vi "5.11-OCU TCP Data Client.vi"() -> ()   [LabVIEW 2010]
doc: "Displays data sent via TCP from Data Server.vi. Once a TCP connection is open, the VI reads 4 bytes to determine the amount of data being sent. It then reads and charts that many bytes. If an error occurs or the stop button is pressed, it sends a \"Q\" to the Data Sender to notify it to quit.\n\n<B>Note:</B> Requires the Data Server.vi located in the same library as this VI."
uses:
  6-OCU Neurons/6.0-OCU to Forebrain Neuron.ctl
  6-OCU Neurons/6.1-Act.ctl
  6-OCU Neurons/6.1-UDP Saitek.ctl
  7-OCU/7.3-Mission Def/7.6 - GPS Waypoint Def.ctl
  6-OCU Neurons/MDF Array LatLong.ctl
  6-OCU Neurons/MDF LatLong.ctl
  5.0-Global.vi
panel:
  in  "Port":u16=22234 min=1025 step=1
  # "Instructions:\n1. Open the Data Server.vi located in the same library.\n2. Follow the instructions on it's front panel.\n\nNote: This VI is built to work with the Data Server.vi."
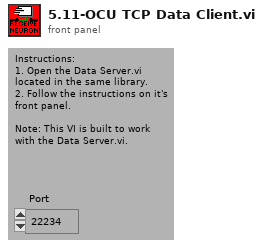
[diagram p1: front panel]
types:
  T1 = typedef "6.0-OCU to Forebrain Neuron.ctl" = cluster{"6.1 Act":T2, "7.6 - GPS Waypoints Data":T4}
  T2 = typedef "6.1-Act.ctl" = cluster{"6.1-Saitek Controller":T3, "Joystick Mode":bool, "Shutdown":bool, "Reset":bool, "Begin":bool}
  T3 = typedef "6.1-UDP Saitek.ctl" = cluster{"Stop":bool, "Setpoint":bool, "Run":bool, "Restart":bool, "Shutdown":bool, "Joystick\nMode 1":bool, "Joystick\nMode 2":bool, "Joystick \nMode 3":bool, "Joystick Mode 4":bool, "10":bool, "11":bool, "Pitch":sgl, "Roll":sgl, "Yaw":sgl, "Left":sgl, "Right":sgl}
  T4 = typedef "7.6 - GPS Waypoint Def.ctl" = cluster{"GPS Waypoint Center (Lat, Long)":dbl[], "5.1.1 MDF GPS":T5}
  T5 = typedef "MDF Array LatLong.ctl" = T6[]
  T6 = typedef "MDF LatLong.ctl" = cluster{"Waypoint #":dbl, "Latitude (waypoint)":ext, "Longitude  (waypoint)":ext}
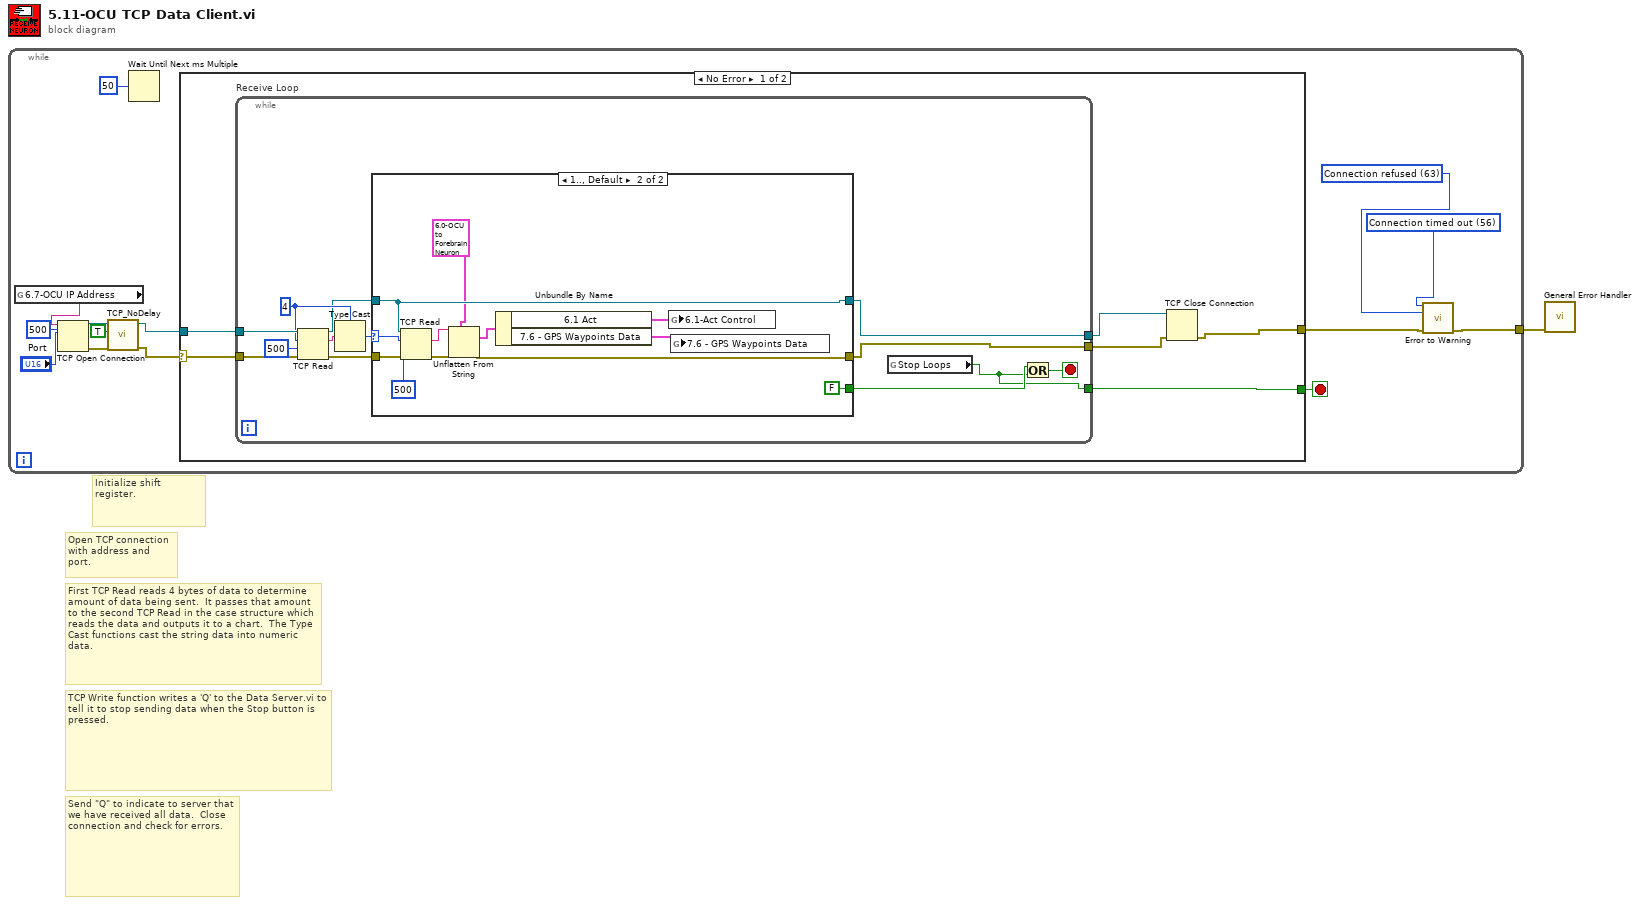
[diagram p0: block diagram]
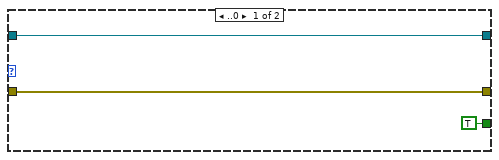
[diagram p2: hidden frame]
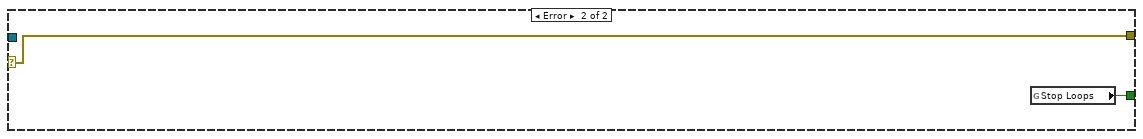
[diagram p3: hidden frame]
diagram:
  # "Initialize shift register."
  # "Send \"Q\" to indicate to server that we have received all data.  Close connection and check for errors."
  # "TCP Write function writes a 'Q' to the Data Server.vi to tell it to stop sending data when the Stop button is pressed."
  # "First TCP Read reads 4 bytes of data to determine amount of data being sent.  It passes that amount to the second TCP Read in the case structure which reads the data and outputs it to a chart.  The Type Cast functions cast the string data into numeric data."
  # "Open TCP connection with address and port."
  n1 = while {
    tunnel: [w5] -> w1
    stop <- w14 stop-if-true
    w3 = 63 items=["No Error", "Argument Error", "Memory Full", "Out of Zone", "End of File", "File Already Open", "Generic File IO Error", "File Not Found", "File Permission Error", "Disk Full", "Duplicate Path", "Too Many Files Open", "Not Enabled", "Resource File Not Found", "Cannot Add Resource", "Resource Not Found", "Image Not Found", "Image Memory Error", "Pen Does Not Exist", "Config Bad Type", "Config Token Not Found", "Config Parse Error", "Config Memory Error", "Bad External Code Format", "Bad External Code Offset", "External Code Not Present", "Null Window", "Destroy Window Mixup", "Null Menu", "Print Aborted", "Bad Print Record", "Print Driver Error", "Windows Error During Print", "Memory Error During Print", "Print Dialog Error", "Generic Print Error", "Invalid Device Refnum", "Device Not Found", "Device Parameter Error", "Device Unit Error", "Can't Open Device", "Device Call Aborted", "Generic Error", "Cancelled By User", "Object ID Too Low", "Object ID Too High", "Object Not In Heap", "Unknown Heap", "Bad DefProc ID", "DefProc Not In Table", "Message Out Of Range", "Null Method", "Unknown Message", "Manager Call Not Supported", "Bad address", "Connection In progress", "Connection timed out", "Connection is already in progress", "Network attribute not supported", "Network error", "Address in use", "System out of memory", "Connection aborted", "Connection refused", "Connection is not connected", "Connection is already connected", "Connection closed", "Initialize error (interapplication manager)", "Bad occurrence", "Wait on unbound occurrence handler", "Occurrence queue overflow", "Bad path", "Semaphore not signaled", "Unrecognized type (interapplication manager)"] ("3rd Error to Convert")
    w4 = 56 items=["No Error", "Argument Error", "Memory Full", "Out of Zone", "End of File", "File Already Open", "Generic File IO Error", "File Not Found", "File Permission Error", "Disk Full", "Duplicate Path", "Too Many Files Open", "Not Enabled", "Resource File Not Found", "Cannot Add Resource", "Resource Not Found", "Image Not Found", "Image Memory Error", "Pen Does Not Exist", "Config Bad Type", "Config Token Not Found", "Config Parse Error", "Config Memory Error", "Bad External Code Format", "Bad External Code Offset", "External Code Not Present", "Null Window", "Destroy Window Mixup", "Null Menu", "Print Aborted", "Bad Print Record", "Print Driver Error", "Windows Error During Print", "Memory Error During Print", "Print Dialog Error", "Generic Print Error", "Invalid Device Refnum", "Device Not Found", "Device Parameter Error", "Device Unit Error", "Can't Open Device", "Device Call Aborted", "Generic Error", "Cancelled By User", "Object ID Too Low", "Object ID Too High", "Object Not In Heap", "Unknown Heap", "Bad DefProc ID", "DefProc Not In Table", "Message Out Of Range", "Null Method", "Unknown Message", "Manager Call Not Supported", "Bad address", "Connection In progress", "Connection timed out", "Connection is already in progress", "Network attribute not supported", "Network error", "Address in use", "System out of memory", "Connection aborted", "Connection refused", "Connection is not connected", "Connection is already connected", "Connection closed", "Initialize error (interapplication manager)", "Bad occurrence", "Wait on unbound occurrence handler", "Occurrence queue overflow", "Bad path", "Semaphore not signaled", "Unrecognized type (interapplication manager)"] ("1st Error to Convert")
    n2 = global read "5.0-Global.vi" "6.7-OCU IP Address"() -> (w9:string)
    n3 = TCP Open Connection(address=w9, remote port or service name="Port", timeout ms (60000)=500) -> (connection ID=w12:refnum<k5>, error out=w11:errorcluster)  [unwired: 1 in, 1 out]
    n4 = call "TCP_NoDelay.vi"("error in (no error)"=w11, "TCP_NODELAY (true)"=TRUE, "connID"=w12) -> ("error out"=w7:errorcluster, "connID 2"=w8:refnum<k5>)  [unwired: 3 in]
    n5 = Wait Until Next ms Multiple(millisecond multiple=u32 50) -> ()  [unwired: 1 out]
    n6 = case shown="No Error" w7 {
      selector: w7 -> [w21 w50]
      tunnel: w8 -> [w20 _]
      tunnel: [w19 w51] -> w14
      tunnel: [w16 w50] -> w6
      frame No Error {
        n7 = while "Receive Loop" {
          tunnel: w21 -> [w32]
          tunnel: w20 -> [w33]
          tunnel: [w23] -> w19
          tunnel: [w27] -> w18
          tunnel: [w26] -> w17
          stop <- w25 stop-if-true
          w31 = 4
          n8 = TCP Read(connection ID=w33, bytes to read=w31, error in (no error)=w32, 9:500 ("timeout ms (25000)")) -> (connection ID out=w28:refnum<k5>, data out=w34:string, error out=w29:errorcluster)  [unwired: 1 out]
          n9 = Type Cast(type=w31, x=w34) -> (*(type *) &x=w30:i32)
          n10 = case shown="1.., Default" w30 {
            selector: w30 -> [_ w48]
            tunnel: w29 -> [w35 w49]
            tunnel: w28 -> [w37 w44]
            tunnel: [w37 w44] -> w27
            tunnel: [TRUE FALSE] -> w24
            tunnel: [w35 w43] -> w26
            frame ..0 {
            }
            frame 1.., Default {
              n11 = TCP Read(connection ID=w44, bytes to read=w48, error in (no error)=w49, 9:500 ("timeout ms (25000)")) -> (data out=w45:string, error out=w46:errorcluster)  [unwired: 2 out]
              n12 = Unflatten From String(type=T1 {"6.1 Act"={"6.1-Saitek Controller"={"Stop"=FALSE, "Setpoint"=FALSE, "Run"=FALSE, "Restart"=FALSE, "Shutdown"=FALSE, "Joystick\nMode 1"=FALSE, "Joystick\nMode 2"=FALSE, "Joystick \nMode 3"=TRUE, "Joystick Mode 4"=FALSE, "10"=FALSE, "11"=FALSE, "Pitch"=0.0019531846, "Roll"=-0.0019531846, "Yaw"=-0.007812738, "Left"=0.828135, "Right"=0.81250954}, "Joystick Mode"=FALSE, "Shutdown"=FALSE, "Reset"=FALSE, "Begin"=FALSE}, "7.6 - GPS Waypoints Data"={"GPS Waypoint Center (Lat, Long)"=[], "5.1.1 MDF GPS"=[]}} ("input cluster"), binary string=w45, error in (no error)=w46) -> (value=w40:T1, error out=w43:errorcluster)  [unwired: 2 in, 1 out]
              n13 = Unbundle By Name(w40) -> ("6.1 Act"=w39:T2, "7.6 - GPS Waypoints Data"=w38:T4)
              n14 = global write "5.0-Global.vi" "6.1-Act Control"(w39) -> ()
              n15 = global write "5.0-Global.vi" "7.6 - GPS Waypoints Data"(w38) -> ()
            }
          }
          n16 = global read "5.0-Global.vi" "Stop Loops"() -> (w23:bool)
          n17 = Or(x=w24, y=w23) -> (x .or. y?=w25:bool)
        }
        n18 = TCP Close Connection(connection ID=w18, error in (no error)=w17) -> (error out=w16:errorcluster)  [unwired: 2 out]
      }
      frame Error {
        n19 = global read "5.0-Global.vi" "Stop Loops"() -> (w51:bool)
      }
    }
    n20 = call <vilib>:"Error to Warning.vi"("1st Error to Convert"=w4, "2nd Error to Convert"=w3, "error in"=w6) -> ("warning out"=w5:errorcluster)  [unwired: 12 in]
  }
  n21 = call <vilib>:"General Error Handler.vi"("error in (no error)"=w1) -> ()  [unwired: 1 in, 14 out]
